vi "LV to DAT 1D.vi"(4 "append to file? (new file:F)":bool, 6 "wavenames (.Vx, etc)":string[](array[string]), 7 "filename":string, 8 "error in":errorcluster, 9 "Data":dbl[](array[numeric]), 10 "Comments":string, 11 "path":path) -> (0 "error out":errorcluster, 3 "new file path":path)   [LabVIEW 2016, in "LVtoITX.lvclass"]
uses:
  LVtoITX.lvclass
  Typedefs/Filetype--enum.ctl
  <vilib>/Utility/file.llb/Write Delimited Spreadsheet (string).vi
panel:
  out "appended array":string[][](array[string])
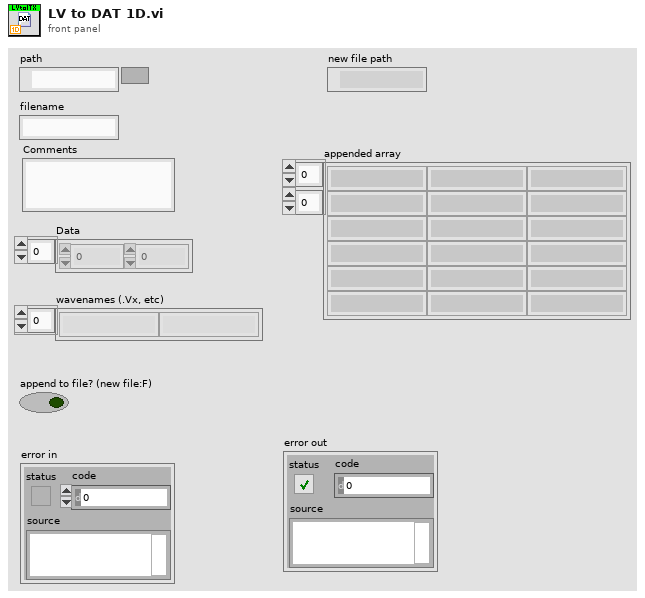
[diagram p1: front panel]
types:
  T1 = typedef "LVtoITX.lvclass/Filetype--enum.ctl" = enum16{"TDMS", "ITX", "DAT"}
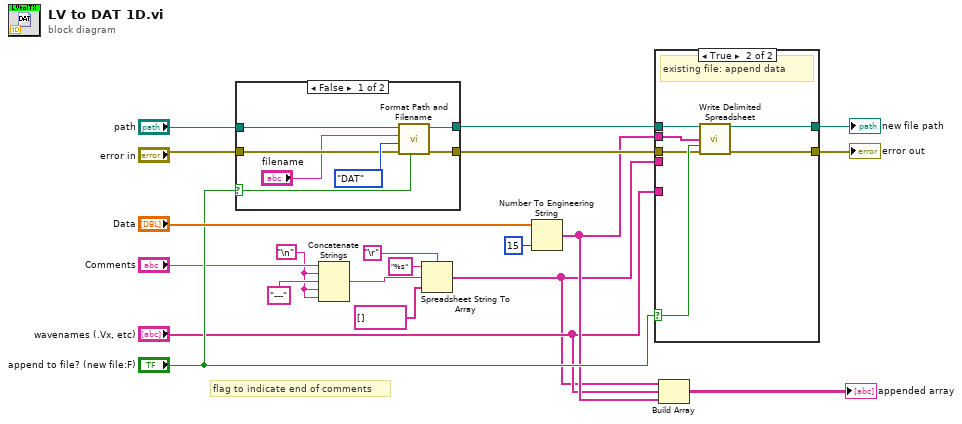
[diagram p0: block diagram]
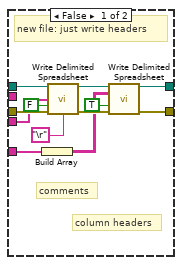
[diagram p3: hidden frame]
diagram:
  w6 = "\n"
  # "flag to indicate end of comments"
  n1 = case shown="False" "append to file? (new file:F)" {
    selector: "append to file? (new file:F)" -> [w27 _]
    tunnel: [w22 w29] -> w20
    tunnel: "path" -> [w23 w29]
    tunnel: "error in" -> [w25 w28]
    tunnel: [w21 w28] -> w14
    frame False {
      n2 = call "Format Path and Filename.vi"("append? (F)"=w27, "error in"=w25, "Type (TDMS)"=Filetype--enum."DAT", "filename"="filename", "path"=w23) -> ("error out"=w21:errorcluster, "path"=w22:path)  [unwired: 4 in, 1 out]
    }
    frame True {
    }
  }
  n3 = Concatenate Strings("Comments", w6, "---" ("string"), w6, w6) -> (w11:string)
  n4 = Spreadsheet String To Array(delimiter (Tab)="\r", format string="%s", spreadsheet string=w11, array type (2D Dbl)=string[] []) -> (array=w2:string[])
  n5 = Number To Engineering String(2:i16 15 ("precision (6)"), 4:"Data") -> (0:w4:string[])  [unwired: 2 out]
  n6 = case shown="True" "append to file? (new file:F)" {
    selector: "append to file? (new file:F)" -> [_ w46]
    tunnel: w2 -> [w34 _]
    tunnel: [w39 w43] -> w13
    tunnel: w4 -> [_ w45]
    tunnel: w20 -> [w41 w47]
    tunnel: w14 -> [w40 w44]
    tunnel: [w36 w42] -> w12
    tunnel: "wavenames (.Vx, etc)" -> [w33 _]
    frame False {
      # "column headers"
      # "comments"
      # "new file: just write headers"
      n7 = Build Array(w33) -> (w32:string[][])
      n8 = call-poly <vilib>:"Write Delimited Spreadsheet.vi"("file path (dialog if empty)"=w41, "1D data"=w34, "append to file? (new file:F)"=FALSE, "error in (no error)"=w40, "delimiter (\\t)"="\r") -> ("new file path (Not A Path if cancelled)"=w37:path, "error out"=w38:errorcluster)  [unwired: 9 in]
      n9 = call-poly <vilib>:"Write Delimited Spreadsheet.vi"("file path (dialog if empty)"=w37, "2D data"=w32, "append to file? (new file:F)"=TRUE, "error in (no error)"=w38) -> ("new file path (Not A Path if cancelled)"=w39:path, "error out"=w36:errorcluster)  [unwired: 10 in]
    }
    frame True {
      # "existing file: append data"
      n10 = call-poly <vilib>:"Write Delimited Spreadsheet.vi"("file path (dialog if empty)"=w47, "1D data"=w45, "append to file? (new file:F)"=w46, "error in (no error)"=w44) -> ("new file path (Not A Path if cancelled)"=w43:path, "error out"=w42:errorcluster)  [unwired: 10 in]
    }
  }
  "new file path" <- w13
  "error out" <- w12
  n11 = Build Array(w2, "wavenames (.Vx, etc)", w4) -> (→"appended array":string[][])
